vi "Get Q.vi"(8 "error in":errorcluster, 9 "Bandwidth":dbl=150.0, 10 "f_center":dbl=1350.0, 11 "PAS Cell Data in":refnum<class "PAS Cell Data.lvclass">) -> (0 "error out":errorcluster, 3 "PAS Cell Data out":refnum<class "PAS Cell Data.lvclass">)   [LabVIEW 2015, in "PAS Cell Data.lvclass"]
doc: "Obtain the parameters associated with calibration of the resonant frequency of the cell. The parameters include the cell quality, resonant frequency and the location and value of the peak of the resonant frequency signal."
uses:
  PAS Cell Data.lvclass
  PAS Cell Data.lvclass/PAS Cell Data.ctl
  General/Math Utilities.lvlib
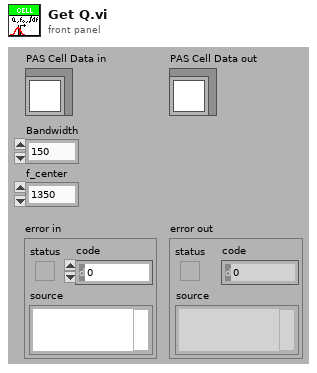
[diagram p1: front panel]
types:
  T1 = typedef "NI_Matrix.lvlib/RealMatrix.ctl" = dbl[][]
  T2 = cluster{"best fit parameters":dbl[], "covariance":T1}
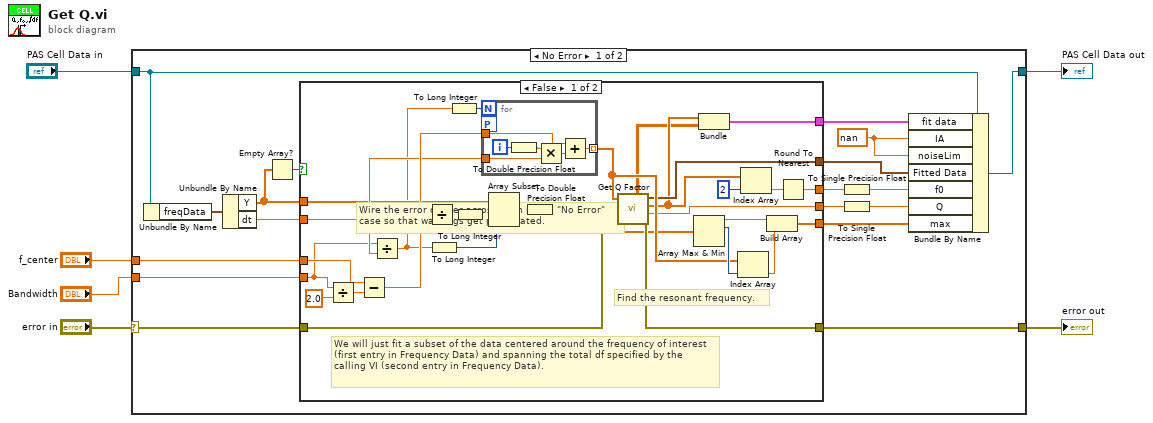
[diagram p0: block diagram]
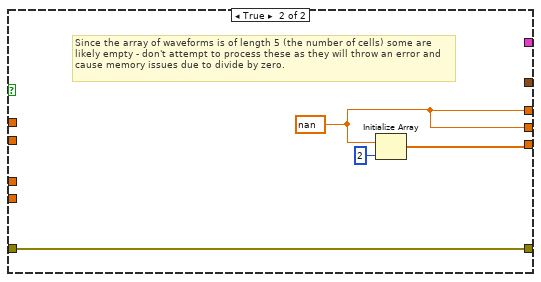
[diagram p2: hidden frame]
diagram:
  n1 = case shown="No Error" "error in" {
    selector: "error in" -> [w20 w65]
    tunnel: [w15 w65] -> w5
    tunnel: [w14 w64] -> w3
    tunnel: "PAS Cell Data in" -> [w19 w64]
    tunnel: "Bandwidth" -> [w8 _]
    tunnel: "f_center" -> [w7 _]
    frame No Error {
      w16 = sgl nan ("IA")
      # "Wire the error cluster across even in the \"No Error\"\ncase so that warnings get propagated."
      n2 = Unbundle By Name(w19) -> ("freqData"=w21:waveform(sgl))
      n3 = Unbundle By Name(w21) -> ("Y"=w24:sgl[], "dt"=w22:dbl)
      n4 = Empty Array?(array=w24) -> (empty?=w23:bool)
      n5 = case shown="False" w23 {
        tunnel: w24 -> [w35 _]
        tunnel: w22 -> [w49 _]
        tunnel: [w48 w63] -> w15
        tunnel: w20 -> [w47 w63]
        tunnel: [w42 _] -> w18
        tunnel: [w33 w60] -> w12
        tunnel: [w41 w60] -> w10
        tunnel: [w40 w61] -> w17
        tunnel: [w37 _] -> w13
        tunnel: w8 -> [w31 _]
        tunnel: w7 -> [w32 _]
        frame False {
          # "Find the resonant frequency."
          # "We will just fit a subset of the data centered around the frequency of interest (first entry in Frequency Data) and spanning the total df specified by the calling VI (second entry in Frequency Data)."
          n6 = Divide(x=w31, y=2.0) -> (x/y=w51:dbl)
          n7 = Subtract ("Floor")(x=w32, y=w51) -> (x-y=w50:dbl)
          n8 = Divide ("Length")(x=w31, y=w49) -> (x/y=w27:dbl)
          n9 = Divide(x=w50, y=w49) -> (x/y=w29:dbl)
          n10 = To Long Integer(number=w27) -> (32bit integer=w26:i32)
          n11 = To Long Integer(number=w27) -> (32bit integer=w36:i32)
          n12 = To Long Integer(number=w29) -> (32bit integer=w28:i32)
          n13 = for {
            N: w36 -> [_]
            tunnel: w50 -> [w59]
            tunnel: w49 -> [w58]
            tunnel: [w56] -> w45 mode=indexing
            workers-P: _ -> [_]
            i -> [w54]
            n14 = To Double Precision Float(number=w54) -> (double precision float=w55:dbl)
            n15 = Multiply(x=w55, y=w58) -> (x*y=w57:dbl)
            n16 = Add(x=w59, y=w57) -> (x+y=w56:dbl)
          }
          n17 = Array Subset(array=w35, index=w28, length=w26) -> (w30:sgl[])
          n18 = To Double Precision Float(number=w30) -> (double precision float=w25:dbl[])
          n19 = call "Get Q Factor.vi"("X"=w45, "Y"=w25, "Error In"=w47) -> ("Fitted Data"=w42:waveform(dbl), "best fit parameters"=w39:dbl[], "Q Factor"=w41:dbl, "error out"=w48:errorcluster, "covariance"=w38:T1)
          n20 = Array Max & Min(array=w25) -> (max value=w44:dbl, max index (indices)=w46:i32)  [unwired: 2 out]
          n21 = Bundle("best fit parameters"=w39, "covariance"=w38) -> (w37:T2)  [unwired: 1 in]
          n22 = Index Array(array=w45, index=w46) -> (element=w43:dbl)
          n23 = Index Array(array=w39, index=2) -> (element=w34:dbl)
          n24 = Build Array(w44, w43) -> (w40:dbl[])
          n25 = Round To Nearest(number=w34) -> (nearest integer value=w33:dbl)
        }
        frame True {
          w60 = nan ("IA")
          # "Since the array of waveforms is of length 5 (the number of cells) some are likely empty - don't attempt to process these as they will throw an error and cause memory issues due to divide by zero."
          n26 = Initialize Array(w60, 2 ("dimension size")) -> (w61:dbl[])
        }
      }
      n27 = To Single Precision Float(number=w12) -> (single precision float=w11:sgl)
      n28 = To Single Precision Float(number=w10) -> (single precision float=w9:sgl)
      n29 = Bundle By Name(cluster=w19, "fit data"=w13, "IA"=w16, "noiseLim"=w16, "Fitted Data"=w18, "f0"=w11, "Q"=w9, "max"=w17) -> (w14:refnum<class "PAS Cell Data.lvclass">)
    }
    frame Error {
    }
  }
  "error out" <- w5
  "PAS Cell Data out" <- w3
